vi "系统交互.vi"   [LabVIEW 2016]
uses:
  <vilib>/Utility/config.llb/NI_LVConfig.lvlib
types:
  T1 = typedef "系统交互.ctl" = cluster{"运行模式":enum16{"维护模式", "常规模式", "应急模式", "质控模式"}, "运行间隔":i16, "流程运行中":bool, "自动运行启动参数":cluster{"氨氮":bool, "总磷总氮":bool, "总氮":bool, "CODmn":bool, "CODCr":bool, "超标留样":bool, "多参数":bool}, "SYSTEM Interface.总磷总氮类型":enum16{"单模块", "二合一模块"}, "多参数运行间隔":i16}
  T2 = cluster{"启动参数":cluster{"氨氮":bool, "总磷":bool, "总氮":bool, "CODMn":bool, "CODCr":bool, "多参数":bool}, "运行模式":enum16{"维护模式", "常规模式", "应急模式", "质控模式"}, "质控频次":enum16{"关闭", "每天", "星期一", "星期二", "星期三", "星期四", "星期五", "星期六", "星期日"}, "空白核查时间":u16, "跨度核查时间":u16, "多参数测试间隔":u16, "湿化学测试间隔":u16}
  T3 = typedef "NI_LVConfig.lvlib/Config Data RefNum.ctl" = refnum<k1>
  T4 = cluster{"氨氮":bool, "总磷总氮":bool, "总氮":bool, "CODmn":bool, "CODCr":bool, "超标留样":bool, "多参数":bool}
  T5 = cluster{"氨氮":bool, "总磷":bool, "总氮":bool, "CODMn":bool, "CODCr":bool, "多参数":bool}
  T6 = typedef "采配水.lvlib/采配水流程.ctl" = u16
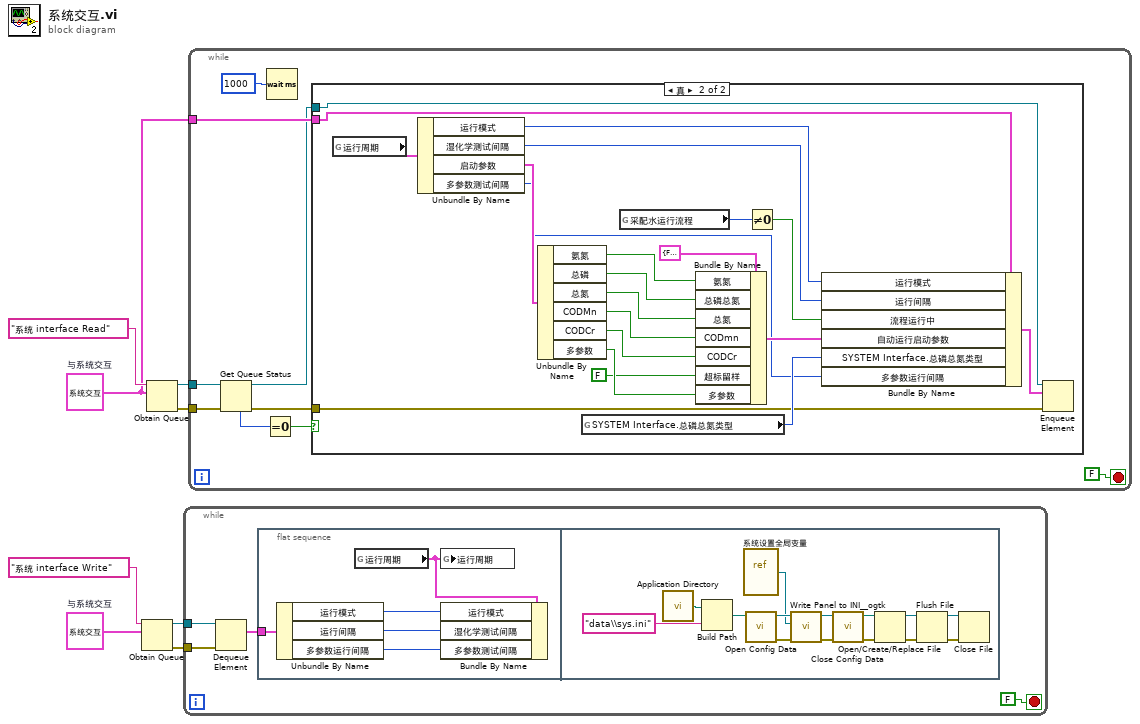
[diagram p0: block diagram]
diagram:
  w4 = T1 {"运行模式"=enum."维护模式", "运行间隔"=4, "流程运行中"=FALSE, "自动运行启动参数"={"氨氮"=FALSE, "总磷总氮"=FALSE, "总氮"=FALSE, "CODmn"=FALSE, "CODCr"=FALSE, "超标留样"=FALSE, "多参数"=FALSE}, "SYSTEM Interface.总磷总氮类型"=enum."单模块", "多参数运行间隔"=4}  # 与系统交互
  w5 = T1 {"运行模式"=enum."维护模式", "运行间隔"=4, "流程运行中"=FALSE, "自动运行启动参数"={"氨氮"=FALSE, "总磷总氮"=FALSE, "总氮"=FALSE, "CODmn"=FALSE, "CODCr"=FALSE, "超标留样"=FALSE, "多参数"=FALSE}, "SYSTEM Interface.总磷总氮类型"=enum."单模块", "多参数运行间隔"=4}  # 与系统交互
  n1 = Obtain Queue(name (unnamed)="系统 interface Write" ("写入方名称"), element data type=w4) -> (queue out=w2:refnum<queue>, error out=w3:errorcluster)  [unwired: 3 in, 1 out]
  n2 = Obtain Queue(name (unnamed)="系统 interface Read" ("写入方名称"), element data type=w5) -> (queue out=w7:refnum<queue>, error out=w6:errorcluster)  [unwired: 3 in, 1 out]
  n3 = while {
    tunnel: w2 -> [w11]
    tunnel: w3 -> [w10]
    stop <- FALSE stop-if-true
    n4 = Dequeue Element(queue=w11, error in (no error)=w10) -> (element=w9:T1)  [unwired: 1 in, 3 out]
    n5 = flat-sequence {
      tunnel: w9 -> [w17]
      frame #0 {
        n6 = Unbundle By Name(w17) -> ("运行模式"=w16:enum16{"维护模式", "常规模式", "应急模式", "质控模式"}, "运行间隔"=w15:i16, "多参数运行间隔"=w14:i16)
        n7 = global read "系统设置全局变量.vi" "运行周期"() -> (w13:T2)
        n8 = global write "系统设置全局变量.vi" "运行周期"(w13) -> ()
        n9 = Bundle By Name(cluster=w13, "运行模式"=w16, "湿化学测试间隔"=w15, "多参数测试间隔"=w14) -> ()  [unwired: 1 out]
      }
      frame #1 {
        n10 = call <vilib>:"Application Directory.vi"() -> ("Application Directory"=w31:path)
        n11 = Build Path(base path=w31, name or relative path="data\\sys.ini" ("名称或相对路径")) -> (appended path=w29:path)
        n12 = vi-ref "系统设置全局变量.vi"() -> (w27:refnum<vi>)
        n13 = call <vilib>:"Open Config Data.vi"("configuration file path"=w29) -> ("error out"=w25:errorcluster, "refnum"=w28:T3)  [unwired: 8 in, 1 out]
        n14 = call <userlib>:"Write Panel to INI__ogtk.vi"("error in (no error)"=w25, "VI ref"=w27, "refnum"=w28) -> ("error out"=w24:errorcluster, "refnum out"=w26:T3)  [unwired: 7 in]
        n15 = call <vilib>:"Close Config Data.vi"("error in (no error)"=w24, "refnum"=w26) -> ("error out"=w19:errorcluster, "file path"=w18:path)  [unwired: 8 in]
        n16 = Open/Create/Replace File(file path (use dialog)=w18, error in=w19) -> (refnum out=w22:refnum<file>, error out=w23:errorcluster)  [unwired: 4 in, 1 out]
        n17 = Flush File(refnum=w22, error in=w23) -> (refnum out=w21:refnum<file>, error out=w20:errorcluster)
        n18 = Close File(refnum=w21, error in=w20) -> ()  [unwired: 2 out]
      }
    }
  }
  n19 = while {
    tunnel: w7 -> [w38]
    tunnel: w6 -> [w34]
    tunnel: w5 -> [w37]
    stop <- FALSE stop-if-true
    n20 = Get Queue Status(queue=w38, error in (no error)=w34) -> (queue out=w36:refnum<queue>, error out=w32:errorcluster, # elements in queue=w35:i32)  [unwired: 1 in, 5 out]
    n21 = Equal To 0?(x=w35) -> (x = 0?=w33:bool)
    n22 = Wait (ms)(milliseconds to wait=u32 1000 ("等待时间（毫秒）")) -> ()  [unwired: 1 out]
    n23 = case shown="真" w33 {
      tunnel: w37 -> [_ w61]
      tunnel: w36 -> [_ w58]
      tunnel: w32 -> [_ w57]
      frame False {
      }
      frame True {
        n24 = global read "系统设置全局变量.vi" "运行周期"() -> (w56:T2)
        n25 = Unbundle By Name(w56) -> ("运行模式"=w55:enum16{"维护模式", "常规模式", "应急模式", "质控模式"}, "湿化学测试间隔"=w54:u16, "启动参数"=w50:T5, "多参数测试间隔"=w41:u16)
        n26 = Unbundle By Name(w50) -> ("氨氮"=w49:bool, "总磷"=w48:bool, "总氮"=w47:bool, "CODMn"=w46:bool, "CODCr"=w45:bool, "多参数"=w44:bool)
        n27 = global read "系统设置全局变量.vi" "SYSTEM Interface.总磷总氮类型"() -> (w60:enum16{"单模块", "二合一模块"})
        n28 = global read "通讯全局变量.vi" "采配水运行流程"() -> (w53:T6)
        n29 = Bundle By Name(cluster=T4 {"氨氮"=FALSE, "总磷总氮"=FALSE, "总氮"=FALSE, "CODmn"=FALSE, "CODCr"=FALSE, "超标留样"=FALSE, "多参数"=FALSE} ("自动运行启动参数"), "氨氮"=w49, "总磷总氮"=w48, "总氮"=w47, "CODmn"=w46, "CODCr"=w45, "超标留样"=FALSE, "多参数"=w44) -> (w42:T4)
        n30 = Not Equal To 0?(x=w53) -> (x != 0?=w52:bool)
        n31 = Bundle By Name(cluster=w61, "运行模式"=w55, "运行间隔"=w54, "流程运行中"=w52, "自动运行启动参数"=w42, "SYSTEM Interface.总磷总氮类型"=w60, "多参数运行间隔"=w41) -> (w59:T1)
        n32 = Enqueue Element(queue=w58, element=w59, error in (no error)=w57) -> ()  [unwired: 1 in, 3 out]
      }
    }
  }
